vi "Result_Test.vi"(8 "error in (no error)":errorcluster caption="entrée d'erreur (pas d'erreur)", 11 "Get_Voltage en entrée":refnum<class "Nodon_Get_FW_Version.lvclass">) -> (0 "error out":errorcluster caption="sortie d'erreur", 3 "Get_Voltage en sortie":refnum<class "Nodon_Get_FW_Version.lvclass">)   [LabVIEW 2020, in "Library Test.lvlib" / "Nodon_Get_FW_Version.lvclass"]
uses:
  Nodon_Get_FW_Version.lvclass
  C:/Users/ngarcin/OneDrive - Altyor/Standard TB/Class/Test/Test (Default)/Test (Default).lvclass
  JSON API/JSON Value/Set from JSON string.vi
  JSON API/JSON Value/JSON Value.lvclass
  Nodon_Send_Command_UART.lvclass
  Nodon_Get_FW_Version.lvclass/Nodon_Get_FW_Version.ctl
  JSON API/Variant JSON/Variant JSON.lvlib
  JSON API/Get Polymorphic/JSON GetSet.lvlib
  Commun VI/Library Commun.lvlib
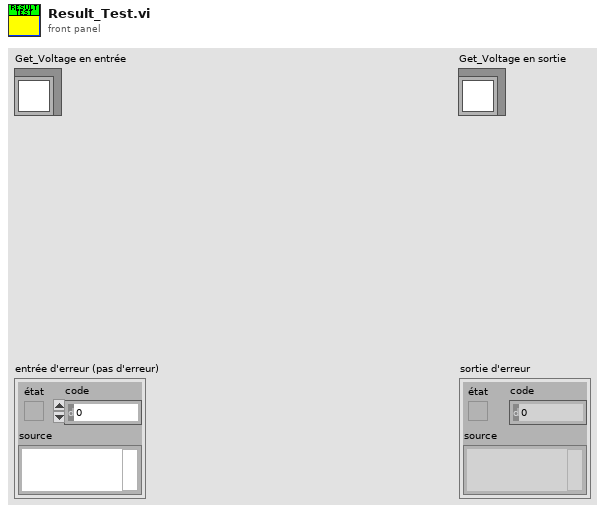
[diagram p1: front panel]
types:
  T1 = cluster{"Commande Type":string, "Command ID":string, "Data":string, "Error":string}
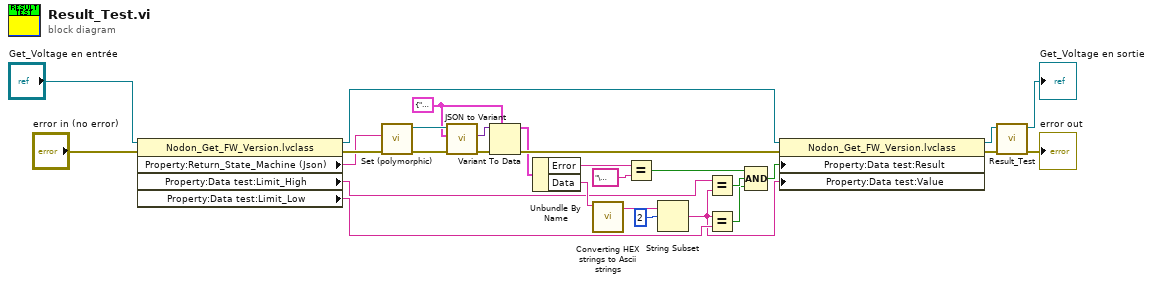
[diagram p0: block diagram]
diagram:
  w12 = T1 {"Commande Type"="", "Command ID"="", "Data"="", "Error"=""}
  n1 = property class="Nodon_Get_FW_Version.lvclass"(reference="Get_Voltage en entrée", error in="error in (no error)") -> (reference out=w26:refnum<class "Nodon_Get_FW_Version.lvclass">, error out=w21:errorcluster, "Property:Return_State_Machine (Json)"=w19:string, "Property:Data test:Limit_High"=w7:string, "Property:Data test:Limit_Low"=w5:string)
  n2 = call-poly "Set (polymorphic).vi"("error in (no error)"=w21, "JSON stream"=w19) -> ("error out"=w23:errorcluster, "JSON Value out"=w25:refnum<class "JSON Value.lvclass">)  [unwired: 7 in, 1 out]
  n3 = call "JSON to Variant.vi"("error in (no error)"=w23, "Variant (Data Type)"=w12, "JSON Value"=w25) -> ("error out"=w24:errorcluster, "Variant out"=w22:variant)  [unwired: 7 in]
  n4 = Variant To Data(error in=w24, type=w12, Variant=w22) -> (data=w18:T1, error out=w20:errorcluster)
  n5 = Unbundle By Name(w18) -> ("Error"=w17:string, "Data"=w10:string)
  n6 = call "Converting HEX strings to Ascii strings.vi"("chaîne IN"=w10) -> ("Chaîne OUT"=w3:string)  [unwired: 9 in, 1 out]
  n7 = Equal?(x=w17, y="\u0000") -> (x = y?=w9:bool)
  n8 = String Subset(string=w3, offset (0)=2) -> (substring=w1:string)  [unwired: 1 in]
  n9 = Equal?(x=w7, y=w1) -> (x = y?=w6:bool)
  n10 = Equal?(x=w1, y=w5) -> (x = y?=w4:bool)
  n11 = Compound Arithmetic op=AND ("Opérateur arithmétique")(w9, w6, w4) -> (w8:bool)
  n12 = property class="Nodon_Get_FW_Version.lvclass"(reference=w26, error in=w20, "Property:Data test:Result"=w8, "Property:Data test:Value"=w1) -> (reference out=w13:refnum<class "Nodon_Get_FW_Version.lvclass">, error out=w11:errorcluster)
  n13 = call-parent "Result_Test.vi"("error in (no error)"=w11, "Get_Voltage en entrée"=w13) -> ("error out"=→"error out":errorcluster, "Get_Voltage en sortie"=→"Get_Voltage en sortie":refnum<class "Nodon_Get_FW_Version.lvclass">)  [unwired: 8 in]
